vi "Create_Analogue_Time_Array.vi"(0 "Sampling Rate (Hz)":dbl, 1 "Sync Delay (s)":dbl, 2 "No of Samples":i32, 3 "Index":i32, 4 "Total No of Chs":i32) -> (5 "Times":dbl[](array[numeric]))   [LabVIEW 2022 SP3]
uses:
  Globals/Meas_global.vi
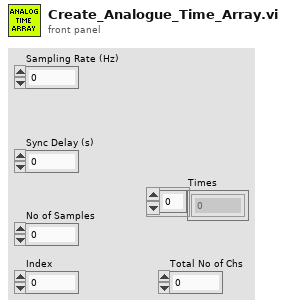
[diagram p1: front panel]
types:
  T1 = typedef "Trigger_Mode.ctl" = enum16{"Free Running", "Start on Trigger", "Trigger Every Block", "Trigger Every Sample"}
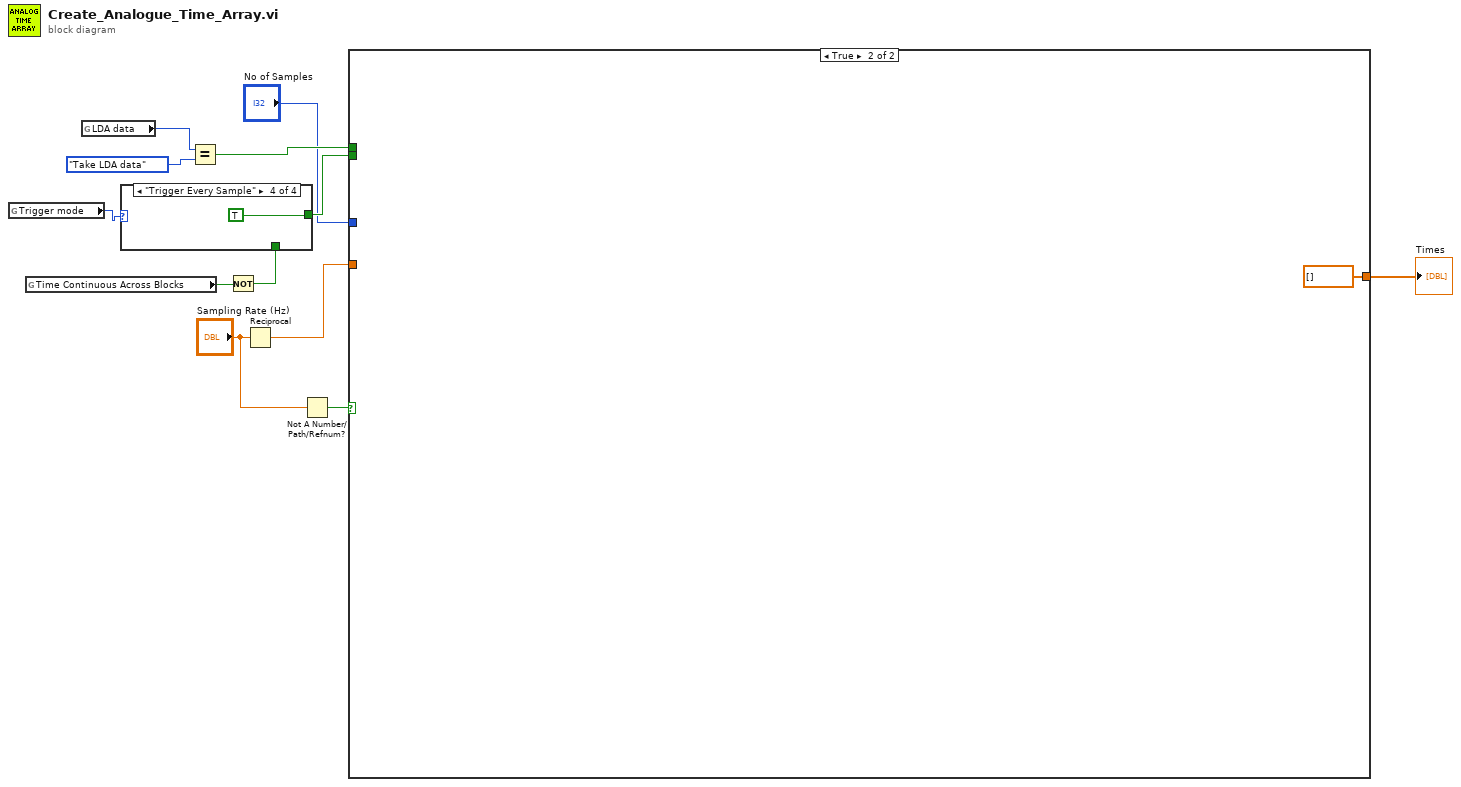
[diagram p0: block diagram]
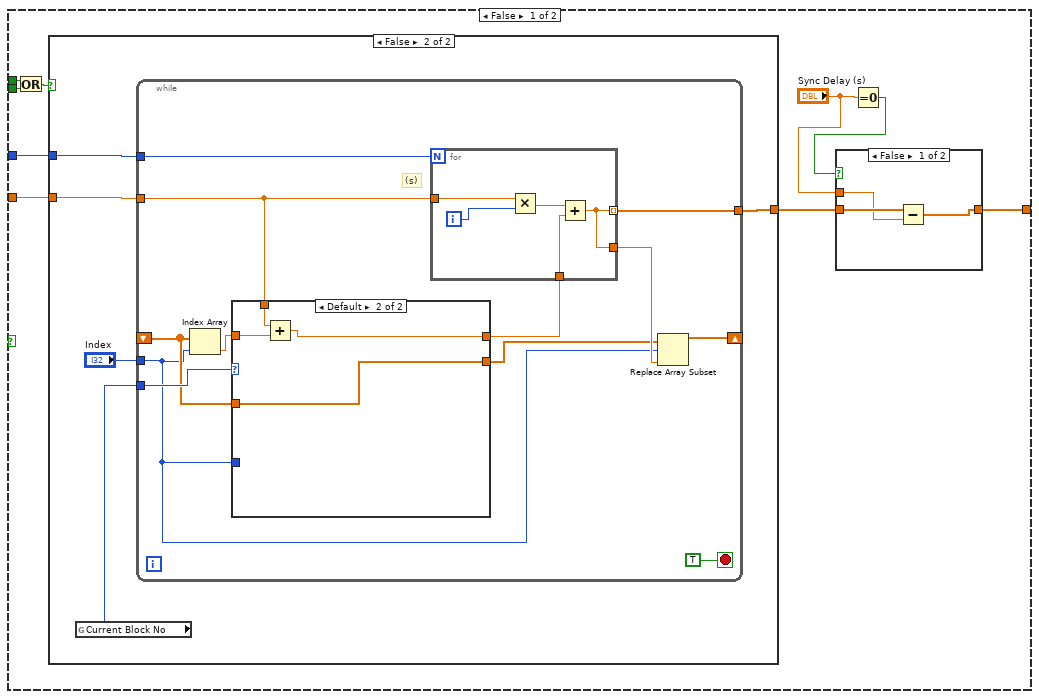
[diagram p2: hidden frame]
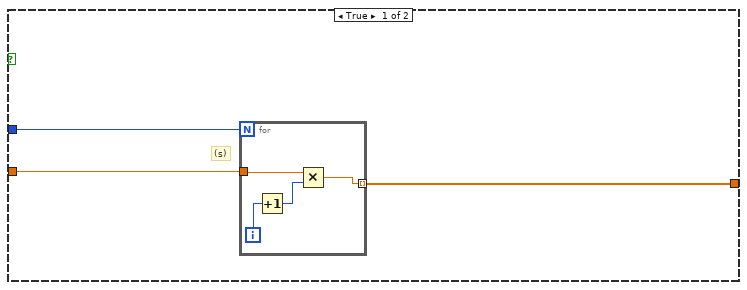
[diagram p4: hidden frame]
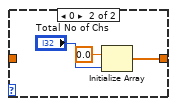
[diagram p6: hidden frame]
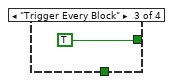
[diagram p9: hidden frame]
diagram:
  n1 = global read "Meas_global.vi" "Trigger mode"() -> (w11:T1)
  n2 = global read "Meas_global.vi" "Time Continuous Across Blocks"() -> (w7:bool)
  n3 = global read "Meas_global.vi" "LDA data"() -> (w5:enum16{"No LDA data", "Take LDA data"})
  n4 = Equal?(x=w5, y=enum16{"No LDA data", "Take LDA data"}."Take LDA data" ("LDA data")) -> (x = y?=w9:bool)
  n5 = Not(x=w7) -> (.not. x?=w6:bool)
  n6 = case shown="\"Trigger Every Sample\"" w11 {
    tunnel: [w13 w14 TRUE TRUE] -> w8
    tunnel: w6 -> [w13 w14 _ _]
    frame "Free Running" {
    }
    frame "Start on Trigger" {
    }
    frame "Trigger Every Block" {
    }
    frame "Trigger Every Sample" {
    }
  }
  n7 = Reciprocal(x="Sampling Rate (Hz)") -> (1/x=w12:dbl)
  n8 = Not A Number/Path/Refnum?(number/path/refnum="Sampling Rate (Hz)") -> (NaN/Path/Refnum?=w2:bool)
  n9 = case shown="True" w2 {
    tunnel: w12 -> [w25 _]
    tunnel: w9 -> [w23 _]
    tunnel: w8 -> [w22 _]
    tunnel: "No of Samples" -> [w21 _]
    tunnel: [w19 dbl[] []] -> w3
    frame False {
      n10 = Or(x=w23, y=w22) -> (x .or. y?=w24:bool)
      n11 = case shown="False" w24 {
        tunnel: [w32 w41] -> w18
        tunnel: w21 -> [w31 w40]
        tunnel: w25 -> [w30 w39]
        frame True {
          # "(s)"
          n12 = for {
            N: w31 -> [_]
            tunnel: w30 -> [w35]
            tunnel: [w34] -> w32 mode=indexing
            i -> [w36]
            n13 = Increment(x=w36) -> (x+1=w33:i32)
            n14 = Multiply(x=w35, y=w33) -> (x*y=w34:dbl)
          }
        }
        frame False {
          n15 = global read "Meas_global.vi" "Current Block No"() -> (w38:i32)
          n16 = while {
            tunnel: [w53] -> w41
            tunnel: w40 -> [w49]
            tunnel: w39 -> [w51]
            shift-right: [w48] -> _
            shift-left: _ -> [w43]
            tunnel: w38 -> [w50]
            tunnel: "Index" -> [w42]
            stop <- TRUE stop-if-true
            # "(s)"
            n17 = Index Array(array=w43, index=w42) -> (element=w46:dbl)
            n18 = case shown="Default" w50 {
              tunnel: [w57 w63] -> w47
              tunnel: w46 -> [_ w65]
              tunnel: w51 -> [w57 w64]
              tunnel: [w56 w62] -> w44
              tunnel: w43 -> [w54 w62]
              tunnel: w42 -> [w55 _]
              frame 1 {
                n19 = case shown="Default" w55 {
                  tunnel: [w58 w59] -> w56
                  tunnel: w54 -> [w58 _]
                  frame Default {
                  }
                  frame 0 {
                    n20 = Initialize Array(0.0 ("element"), "Total No of Chs") -> (w59:dbl[])
                  }
                }
              }
              frame Default {
                n21 = Add(x=w64, y=w65) -> (x+y=w63:dbl)
              }
            }
            n22 = for {
              N: w49 -> [_]
              tunnel: w51 -> [w70]
              tunnel: [w67] -> w53 mode=indexing
              tunnel: w47 -> [w68]
              tunnel: [w67] -> w45
              i -> [w66]
              n23 = Multiply(x=w70, y=w66) -> (x*y=w69:dbl)
              n24 = Add(x=w69, y=w68) -> (x+y=w67:dbl)
            }
            n25 = Replace Array Subset(array=w44, new element=w45, index=w42) -> (w48:dbl[])
          }
        }
      }
      n26 = Equal To 0?(x="Sync Delay (s)") -> (x = 0?=w20:bool)
      n27 = case shown="False" w20 {
        tunnel: [w27 w29] -> w19
        tunnel: w18 -> [w28 w29]
        tunnel: "Sync Delay (s)" -> [w26 _]
        frame False {
          n28 = Subtract(x=w28, y=w26) -> (x-y=w27:dbl[])
        }
        frame True {
        }
      }
    }
    frame True {
    }
  }
  "Times" <- w3
